vi "getRbStrokeFromFile.vi"(8 "error in (no error)":errorcluster, 10 "Rigid Body Stroke File":string="rbStroke.txt", 11 "OptCtrl in":refnum<class "OptCtrl.lvclass">) -> (0 "error out":errorcluster, 2 "Stroke in Um":dbl[](array[numeric]), 3 "OptCtrl out":refnum<class "OptCtrl.lvclass">)   [LabVIEW 2016, in "OptCtrl.lvclass"]
doc: "Get the rigid body stroke from the file. The order is the M2 hexapod followed by the camera hexapod."
uses:
  OptCtrl.lvclass
  OptCtrl.lvclass/OptCtrl.ctl
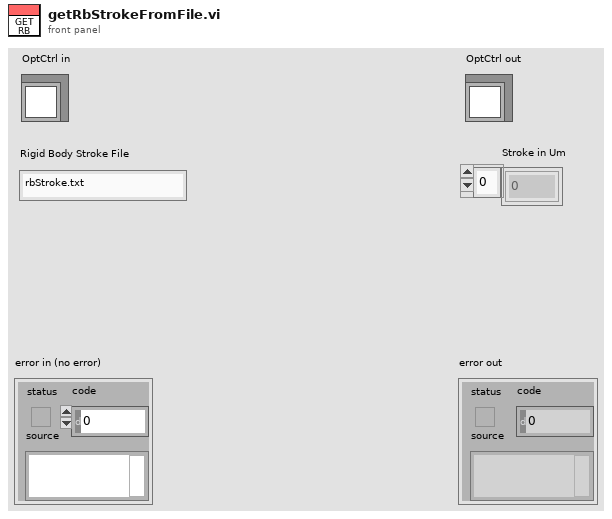
[diagram p1: front panel]
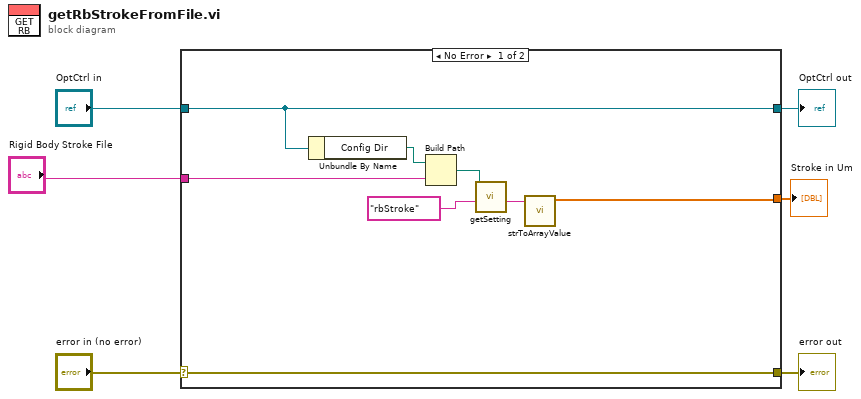
[diagram p0: block diagram]
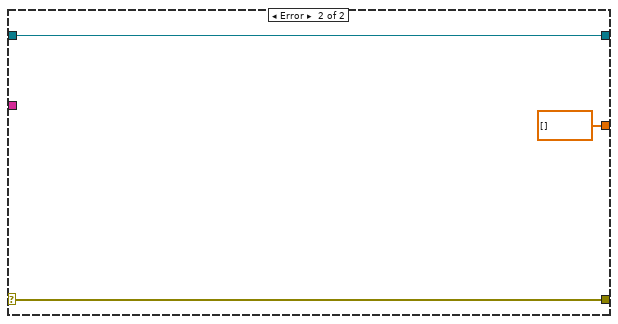
[diagram p2: hidden frame]
diagram:
  n1 = case shown="No Error" "error in (no error)" {
    selector: "error in (no error)" -> [w14 w17]
    tunnel: [w14 w17] -> w5
    tunnel: [w9 w16] -> w3
    tunnel: "OptCtrl in" -> [w9 w16]
    tunnel: "Rigid Body Stroke File" -> [w8 _]
    tunnel: [w7 dbl[] [] ("Array")] -> w1
    frame No Error {
      n2 = Unbundle By Name(w9) -> ("Config Dir"=w13:path)
      n3 = Build Path(base path=w13, name or relative path=w8) -> (appended path=w12:path)
      n4 = call "getSetting.vi"("Parameter"="rbStroke", "Path"=w12) -> ("Value"=w10:string)  [unwired: 8 in, 1 out]
      n5 = call "strToArrayValue.vi"("String"=w10) -> ("Array"=w7:dbl[])  [unwired: 10 in]
    }
    frame Error {
    }
  }
  "error out" <- w5
  "OptCtrl out" <- w3
  "Stroke in Um" <- w1
